vi "Download Package.vi"(8 "error in":errorcluster, 9 "download all dependencies? (T)":bool=TRUE, 10 "destination folder":path, 11 "package name":string) -> (0 "error out":errorcluster)   [LabVIEW 2014, in "NIPM_API.lvlib"]
doc: "Downloads the package and all its dependencies to the destination folder"
uses:
  NIPM_API.lvlib
panel:
  out "cmd standard output":string
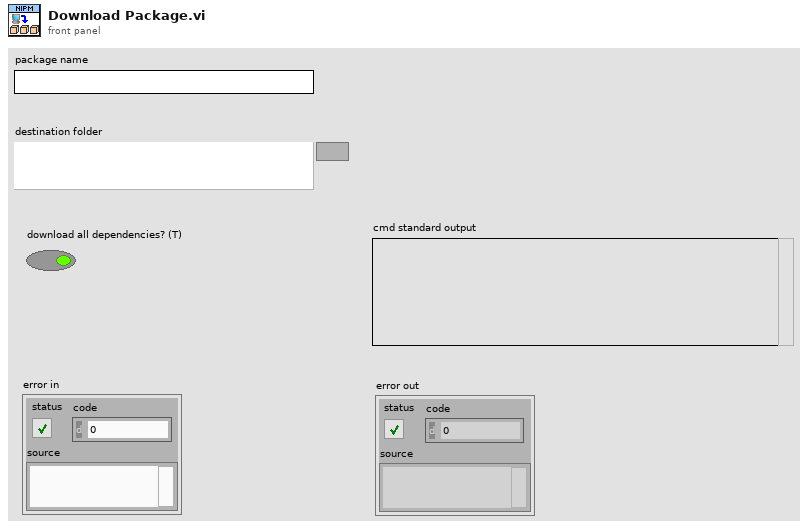
[diagram p1: front panel]
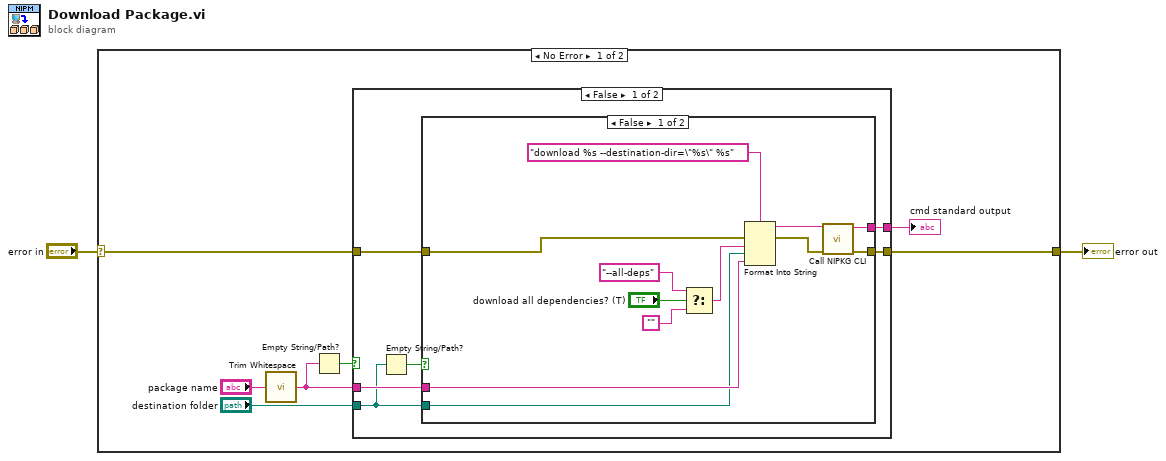
[diagram p0: block diagram]
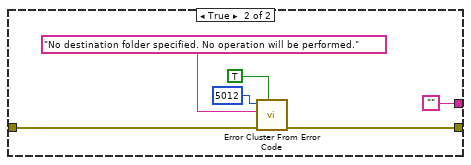
[diagram p2: hidden frame]
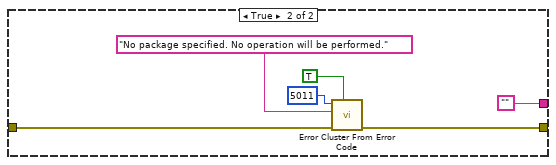
[diagram p3: hidden frame]
diagram:
  n1 = case shown="No Error" "error in" {
    selector: "error in" -> [w9 w40]
    tunnel: [w5 w40] -> w1
    frame No Error {
      n2 = call <vilib>:"Trim Whitespace.vi"("string"="package name") -> ("trimmed string"=w4:string)  [unwired: 1 in]
      n3 = Empty String/Path?(string/path=w4) -> (empty?=w6:bool)
      n4 = case shown="False" w6 {
        tunnel: w9 -> [w15 w35]
        tunnel: "destination folder" -> [w11 _]
        tunnel: w4 -> [w14 _]
        tunnel: [w13 w36] -> w5
        tunnel: [w12 ""] -> w3
        frame False {
          n5 = Empty String/Path?(string/path=w11) -> (empty?=w10:bool)
          n6 = case shown="False" w10 {
            tunnel: w15 -> [w27 w30]
            tunnel: w14 -> [w19 _]
            tunnel: [w18 w29] -> w13
            tunnel: [w17 ""] -> w12
            tunnel: w11 -> [w16 _]
            frame False {
              n7 = Select(t="--all-deps", s="download all dependencies? (T)", f="") -> (s? t:f=w21:string)
              n8 = Format Into String(format string="download %s --destination-dir=\"%s\" %s", error in=w27, w21, w16, w19) -> (resulting string=w26:string, error out=w25:errorcluster)  [unwired: 1 in]
              n9 = call "Call NIPKG CLI.vi"("error in (no error)"=w25, "command"=w26) -> ("error out"=w18:errorcluster, "command line standard output"=w17:string)  [unwired: 8 in]
            }
            frame True {
              n10 = call <vilib>:"Error Cluster From Error Code.vi"("show call chain? (False)"=TRUE, "error in (no error)"=w30, "error message (\"\")"="No destination folder specified. No operation will be performed.", "error code (0)"=5012) -> ("error out"=w29:errorcluster)  [unwired: 5 in]
            }
          }
        }
        frame True {
          n11 = call <vilib>:"Error Cluster From Error Code.vi"("show call chain? (False)"=TRUE, "error in (no error)"=w35, "error message (\"\")"="No package specified. No operation will be performed.", "error code (0)"=5011) -> ("error out"=w36:errorcluster)  [unwired: 5 in]
        }
      }
      "cmd standard output" <- w3
    }
    frame Error {
    }
  }
  "error out" <- w1
